vi "S2DS_Write to external instrument (SubVI).vi"(8 "error in (no error)":errorcluster, 9 "Present value in":dbl, 10 "Target":dbl, 11 "Instrument parameters in":T1) -> (0 "error out":errorcluster, 2 "Present value out":dbl, 3 "Instrument parameters out":T1)   [LabVIEW 2025]
uses:
  TYPE DEFS/S2DS_Instrument parameters.ctl
panel:
  out "Reached?":bool
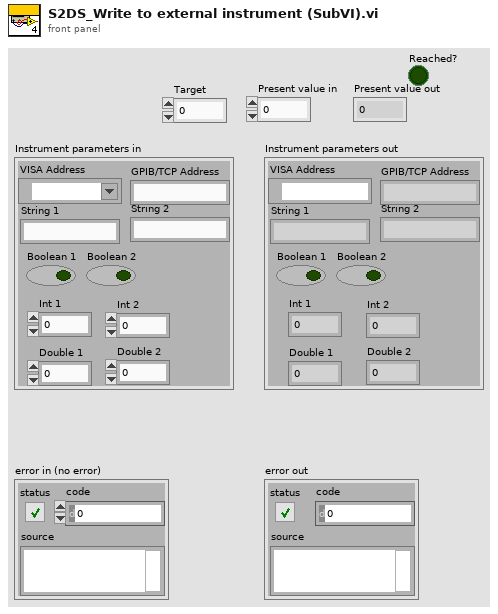
[diagram p1: front panel]
types:
  T1 = typedef "S2DS_Instrument parameters.ctl" = cluster{"VISA Address":refnum<visa-resource-name>, "GPIB/TCP Address":string, "String 1":string, "String 2":string, "Boolean 1":bool, "Boolean 2":bool, "Int 1":i32, "Int 2":i32, "Double 1":dbl, "Double 2":dbl}
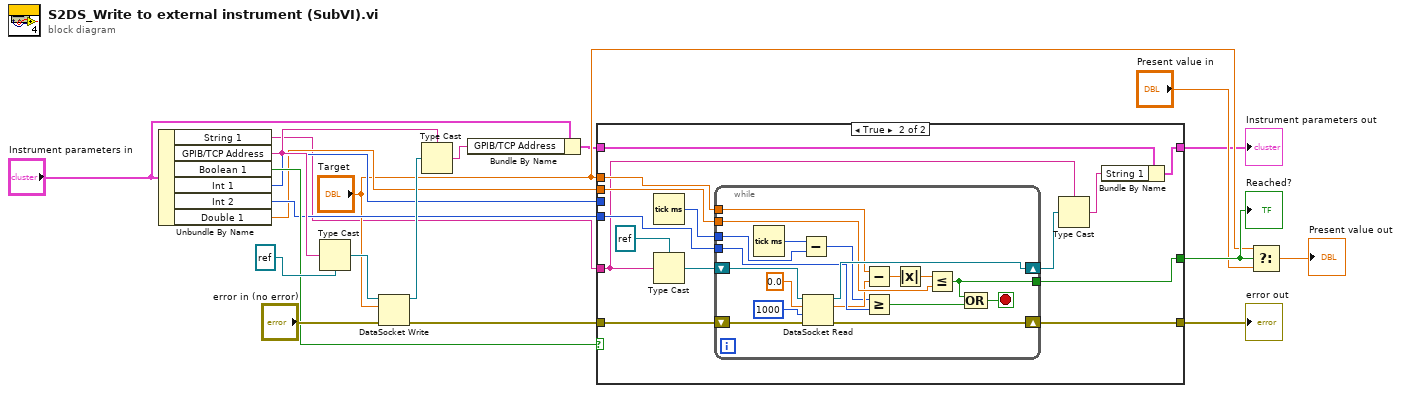
[diagram p0: block diagram]
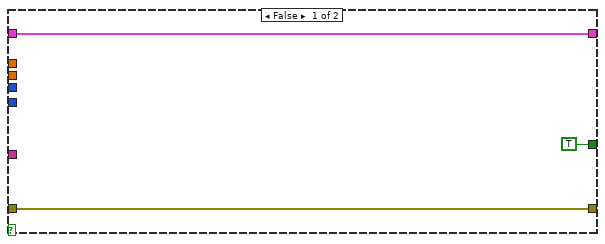
[diagram p2: hidden frame]
diagram:
  n1 = Unbundle By Name("Instrument parameters in") -> ("String 1"=w3:string, "GPIB/TCP Address"=w17:string, "Boolean 1"=w13:bool, "Int 1"=w12:i32, "Int 2"=w9:i32, "Double 1"=w8:dbl)
  n2 = Type Cast(type=refnum<k13> refnum ("connection id"), x=w17) -> (*(type *) &x=w19:refnum<k13>)
  n3 = DataSocket Write(8:"error in (no error)", 10:"Target", 11:w19) -> (0:w11:errorcluster, 3:w16:refnum<k13>)  [unwired: 1 in, 1 out]
  n4 = Type Cast(type=w17, x=w16) -> (*(type *) &x=w14:string)
  n5 = Bundle By Name(cluster="Instrument parameters in", "GPIB/TCP Address"=w14) -> (w2:T1)
  n6 = case shown="True" w13 {
    tunnel: w12 -> [_ _]
    tunnel: w11 -> [w23 w37]
    tunnel: "Target" -> [_ w36]
    tunnel: w8 -> [_ w35]
    tunnel: [w23 w32] -> w10
    tunnel: w9 -> [_ w33]
    tunnel: [TRUE w31] -> w7
    tunnel: w3 -> [_ w27]
    tunnel: w2 -> [w21 w26]
    tunnel: [w21 w24] -> w1
    frame False {
    }
    frame True {
      n7 = Tick Count (ms)() -> (millisecond timer value=w34:u32)
      n8 = Type Cast(type=refnum<k13> refnum ("connection id"), x=w27) -> (*(type *) &x=w29:refnum<k13>)
      n9 = while {
        shift-right: [w54] -> w28
        shift-left: w29 -> [w55]
        shift-right: [w52] -> w32
        shift-left: w37 -> [w53]
        tunnel: w36 -> [w49]
        tunnel: w35 -> [w46]
        tunnel: w34 -> [w44]
        tunnel: w33 -> [w41]
        tunnel: [w38] -> w31
        stop <- w42 stop-if-true
        n10 = Tick Count (ms)() -> (millisecond timer value=w45:u32)
        n11 = Subtract(x=w45, y=w44) -> (x-y=w39:u32)
        n12 = DataSocket Read(8:w53, 9:1000 ("ms timeout (10000)"), 10:0.0, 11:w55) -> (0:w52:errorcluster, 2:w40:dbl, 3:w54:refnum<k13>)  [unwired: 1 in, 4 out]
        n13 = Subtract(x=w49, y=w40) -> (x-y=w48:dbl)
        n14 = Greater Or Equal?(x=w39, y=w41) -> (x >= y?=w43:bool)
        n15 = Absolute Value(x=w48) -> (abs(x)=w47:dbl)
        n16 = Less Or Equal?(x=w47, y=w46) -> (x <= y?=w38:bool)
        n17 = Compound Arithmetic op=OR(w38, w43) -> (w42:bool)
      }
      n18 = Type Cast(type=w27, x=w28) -> (*(type *) &x=w25:string)
      n19 = Bundle By Name(cluster=w26, "String 1"=w25) -> (w24:T1)
    }
  }
  "Instrument parameters out" <- w1
  "error out" <- w10
  "Reached?" <- w7
  n20 = Select(t="Target", s=w7, f="Present value in") -> (s? t:f=→"Present value out":dbl)
